vi "fft_kf_update.vi"(9 "Measurement":cdb[](array[numeric]), 10 "Measure noise covariance":dbl[](array[numeric]), 11 "KF in":T1 {"K" format="%#_3g"; "y lim" format="%#_3g"; "x lim" format="%#_3g"; "P" format="%#_3g"; "H" format="%#_3g"; "x" format="%#_3g"; "Q" format="%#_3g"; "R" format="%#_3g"; "B" format="%#_3g"; "A" format="%#_3g"}) -> (2 "KF out":T1 {"K" format="%#_3g"; "y lim" format="%#_3g"; "x lim" format="%#_3g"; "P" format="%#_3g"; "H" format="%#_3g"; "x" format="%#_3g"; "Q" format="%#_3g"; "R" format="%#_3g"; "B" format="%#_3g"; "A" format="%#_3g"}, 3 "KF estimate":cdb[](array[numeric]))   [LabVIEW 2014]
uses:
  utilities/kalman_filter.ctl
  <vilib>/Analysis/Matrix/Datatypes/RealMatrix.ctl
  <vilib>/Analysis/Matrix/Numeric/Conversions/Array To Matrix - RA2.vi
  <vilib>/Analysis/Matrix/NI_Matrix.lvlib
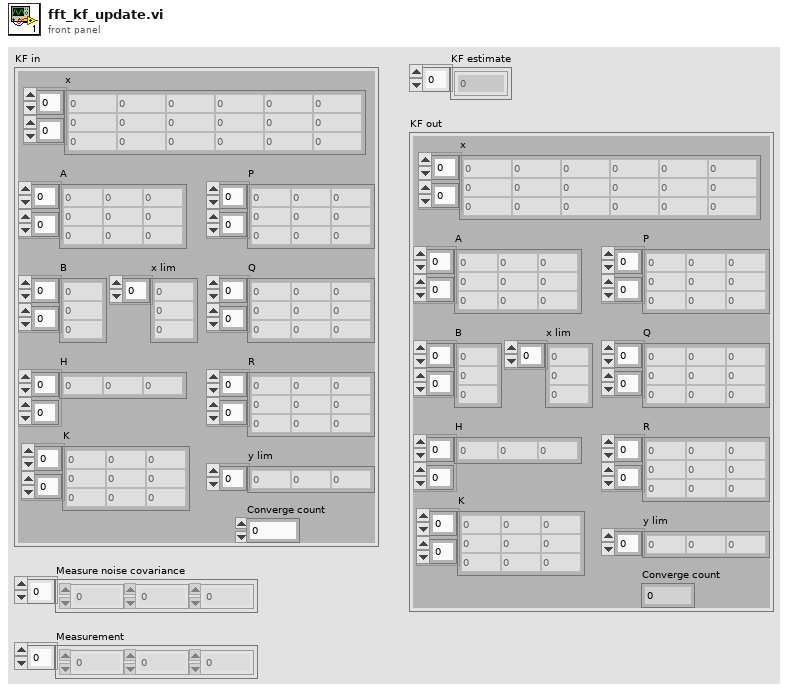
[diagram p1: front panel]
types:
  T1 = typedef "kalman_filter.ctl" = cluster{"A":T2, "B":T2, "H":T2, "Q":T2, "R":T2, "x":T2, "P":T2, "x lim":dbl[], "y lim":dbl[], "K":T2, "Converge count":i32}
  T2 = typedef "NI_Matrix.lvlib/RealMatrix.ctl" = dbl[][]
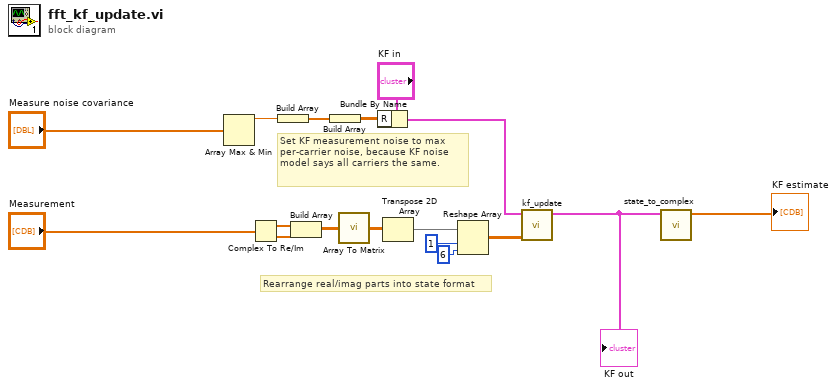
[diagram p0: block diagram]
diagram:
  # "Rearrange real/imag parts into state format"
  # "Set KF measurement noise to max per-carrier noise, because KF noise model says all carriers the same."
  n1 = Array Max & Min(array="Measure noise covariance") -> (max value=w10:dbl)  [unwired: 3 out]
  n2 = Complex To Re/Im(x + iy="Measurement") -> (x=w3:dbl[], y=w4:dbl[])
  n3 = Build Array(w10) -> (w6:dbl[])
  n4 = Build Array(w3, w4) -> (w12:dbl[][])
  n5 = Build Array(w6) -> (w7:T2)
  n6 = call-poly <vilib>:"Array To Matrix.vi"("Real 2D Array"=w12) -> ("Real Matrix"=w13:T2)
  n7 = Bundle By Name(cluster="KF in", "R"=w7) -> (w8:T1)
  n8 = Transpose 2D Array(2D array=w13) -> (transposed array=w11:T2)
  n9 = Reshape Array(w11, 1 ("dimension size"), 6 ("dimension size")) -> (w16:T2)
  n10 = call "kf_update.vi"("z"=w16, "KF in"=w8) -> ("KF out"=w1:T1)  [unwired: 8 in, 1 out]
  "KF out" <- w1
  n11 = call "state_to_complex.vi"("KF in"=w1) -> ("Amplitudes"=→"KF estimate":cdb[])  [unwired: 10 in]
